vi "AR.Drone MAIN.vi"() -> ()   [LabVIEW 2014]
doc: "Very simple example showing how to use the base VIs to control the AR Drone and receive and display video data."
uses:
  Resources/Others/Control cluster.ctl
  <vilib>/LVH/AR Drone Toolkit/Decode NavData/Typedefs/NavData Demo.ctl
  Resources/Global.vi
  <vilib>/LVH/AR Drone Toolkit/AR Drone.lvlib
panel:
  in  "Tab Control 2":enum32{"Setup", "Debug&Test Info", "NavData"}(tab)
  in  "Secondary VI":u16(ring) items=["Auto Hovering with Position Prediction.vi", "Simple Video.vi", "Circle detection.vi", "OCR Control.vi", "", ""]
  in  "Setup Parameters":T1={"Drone IP address"="192.168.1.1", "Home IP address"="192.168.1.2", "Flight Mode"=enum."INDOOR MODE", "Mounted Hull"=enum."INDOOR HULL", "Video Camera"=1, "Max Altitude (m)"=3.0, "Max Pitch and Roll Angle (deg)"=8.0, "Max Vertical Speed (m/s)"=0.7, "Max Yaw Speed (deg/s)"=100.0} {"Video Camera" items=["Bottom Camera"=1, "Front Camera"=0, "Front in Bottom"=3, "Bottom in Front"=2]}
  in  "Controller ID":i32=2
  in  "Adjustments":cluster{"Sensitivity":dbl, "Null Zone":dbl}={"Sensitivity"=1.0, "Null Zone"=1.0} {"Null Zone" scale=0.0..2.0; "Sensitivity" scale=0.0..2.0}
  out "In. device":T2={"axes total"=0, "buttons total"=1280, "pov total"=0, "device name"="Micr"}
  out "Loop iteration":i32=255
  in  "milliseconds to wait":u32=10
  out "Refesh Rate (ms)":u32=10
  out "Refesh Rate Video Loop (ms) 2":u32=40
  in  "video refresh (ms)":u32=40
  out "Error":errorcluster
  out "NavData Out":T3={"control state"=enum."TRANS_LANDING", "battery percentage"=55, "pitch (deg)"=0.026, "roll (deg)"=-0.043, "yaw (deg)"=74.079, "altitude (cm)"=0, "vx (cm/s)?"=0.0, "vy (cm/s)?"=0.0, "vz (cm/s)?"=0.0, "detection cam type"=3}
  out "Battery Remaining":dbl(slide)=55.0 scale=0.0..100.0
  out "Hover":bool
  out "Control Cluster":T4 {"Yaw Speed" scale=-1.0..1.0; "Vertical Speed" scale=-1.0..1.0; "Pitch" scale=-1.0..1.0; "Roll" scale=-1.0..1.0}
  out "error":bool
  out "Take off/Land":bool
  in  "Tab Control":enum32{"Raw Image", "Grayscale", "Black&White"}(tab)=enum."Black&White"
  out "Raw":picture
  out "Grayscale":T5(plugin-control)
  out "B&W":T5(plugin-control)
  in  "Manual":bool=TRUE
  in  "stop":bool
  in  "Emergency Landing":bool
  # "(1 is default)"
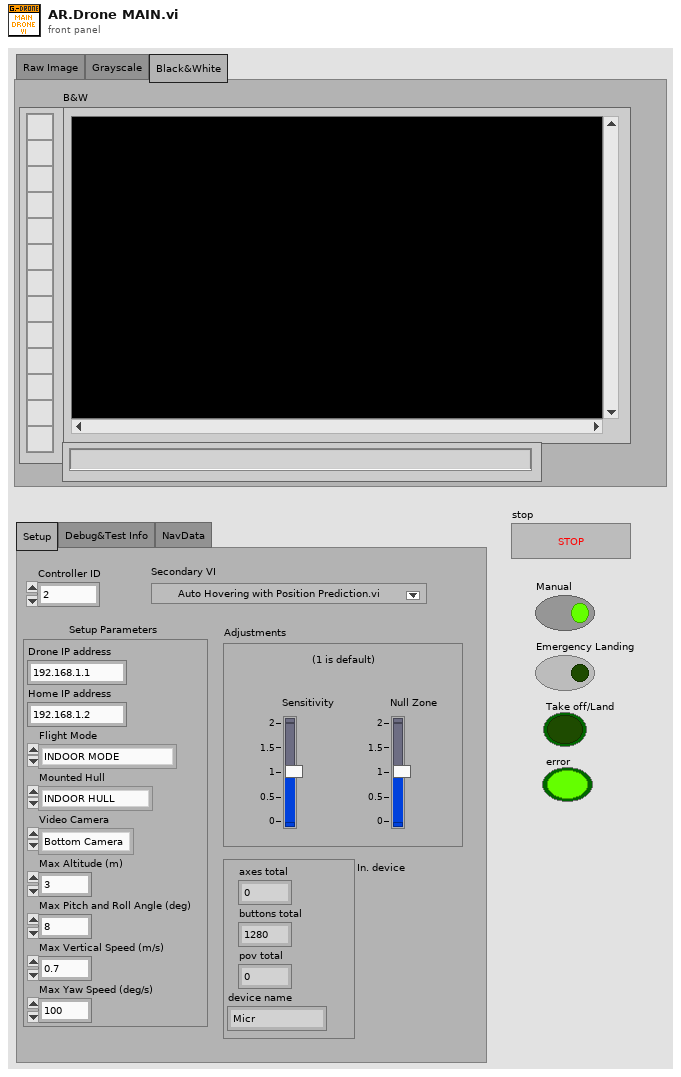
[diagram p1: front panel]
types:
  T1 = cluster{"Drone IP address":string, "Home IP address":string, "Flight Mode":enum8{"OUTDOOR MODE", "INDOOR MODE"}, "Mounted Hull":enum8{"OUTDOOR HULL", "INDOOR HULL"}, "Video Camera":u8, "Max Altitude (m)":sgl, "Max Pitch and Roll Angle (deg)":sgl, "Max Vertical Speed (m/s)":sgl, "Max Yaw Speed (deg/s)":sgl}
  T2 = cluster{"axes total":u32, "buttons total":u32, "pov total":u32, "device name":string}
  T3 = typedef "AR Drone.lvlib/NavData Demo.ctl" = cluster{"control state":enum32{"DEFAULT", "INIT", "LANDING", "FLYING", "HOVERING", "TEST", "TRANS_TAKEOFF", "TRANS_GOTOFIX", "TRANS_LANDING"}, "battery percentage":u32, "pitch (deg)":sgl, "roll (deg)":sgl, "yaw (deg)":sgl, "altitude (cm)":u32, "vx (cm/s)?":sgl, "vy (cm/s)?":sgl, "vz (cm/s)?":sgl, "detection cam type":u32}
  T4 = typedef "Control cluster.ctl" = cluster{"Roll":sgl, "Pitch":sgl, "Vertical Speed":sgl, "Yaw Speed":sgl}
  T5 = typedef "IMAQ Image.ctl" = refnum<image>
  T6 = typedef "AR Drone.lvlib/AR Drone Resource.ctl" = cluster{"UDP Control Connection":refnum<k16>, "UDP NavData Connection":refnum<k16>, "UDP Video Connection (Drone 1.0)":refnum<k16>, "TCP Video Connection (Drone 2.0)":refnum<k5>, "TCP Control Port Connection":refnum<k5>, "Drone IP address":string, "Drone Command Port":u16, "Drone NavData Port":u16, "Drone Vid Stream Port":u16, "Drone TCP Control Port":u16, "Home IP address":string, "Home Command Port":u16, "Home NavData Port":u16, "Home Vid Stream Port":u16, "Drone Version":i32, "Drone Index":i32, "Command Sequence":i32}
  T7 = cluster{"Roll":dbl, "Pitch":dbl, "Vertical Speed":dbl, "Yaw Speed":dbl}
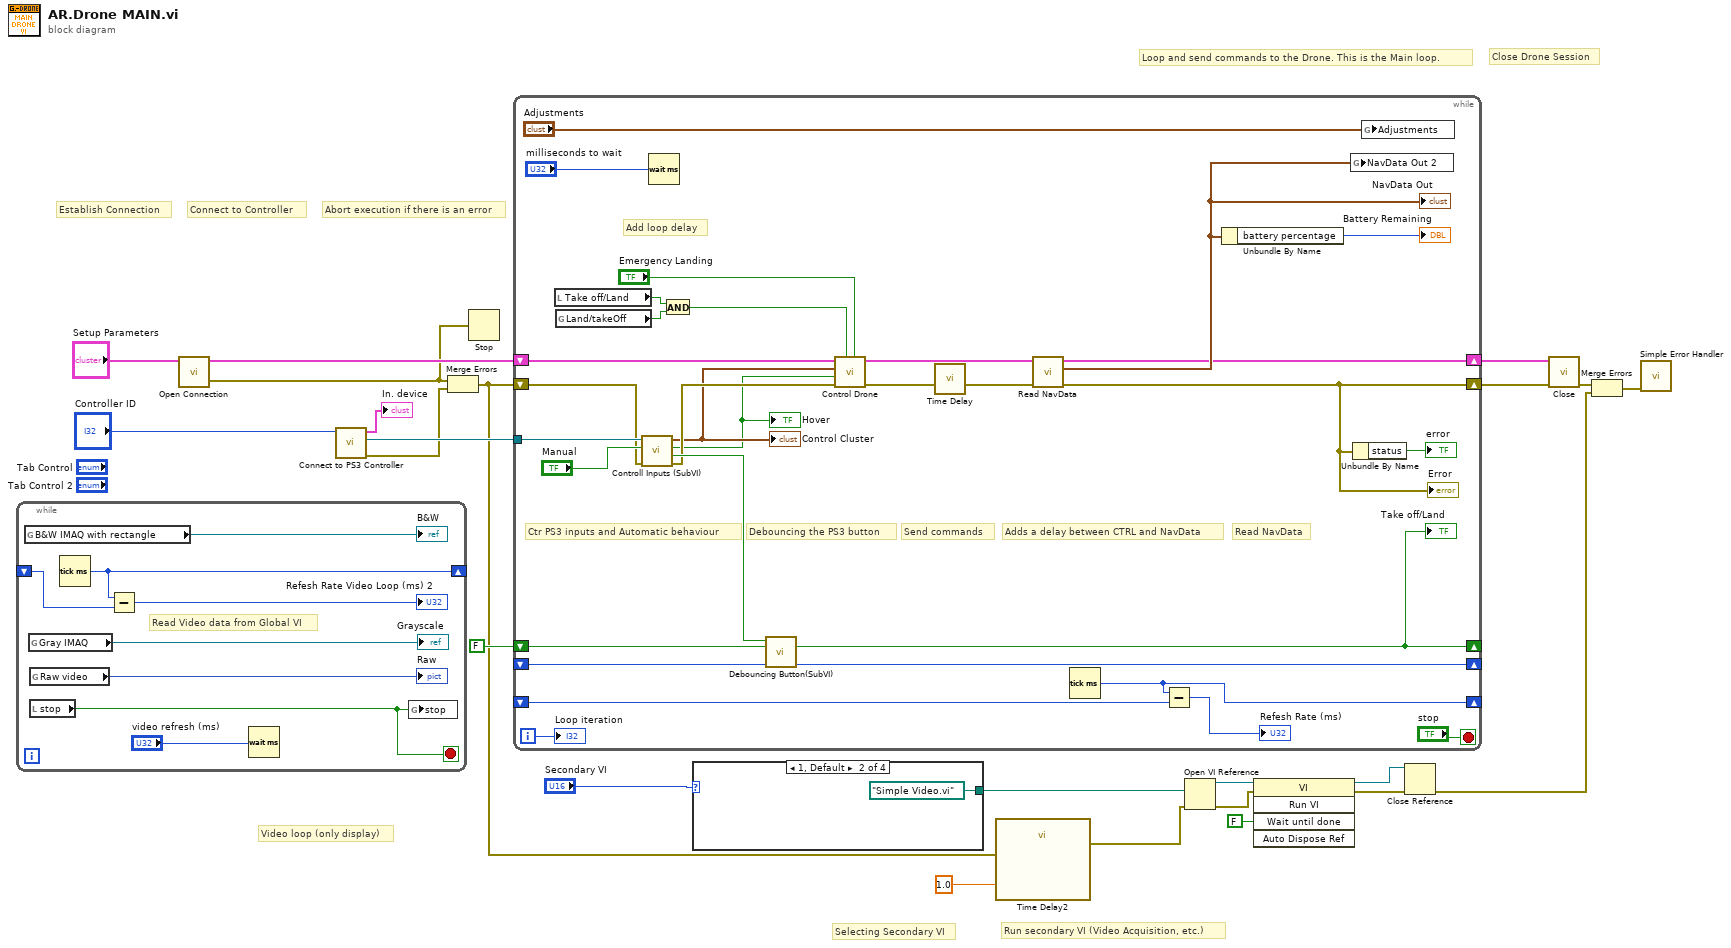
[diagram p0: block diagram]
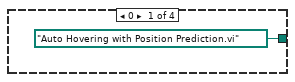
[diagram p2: hidden frame]
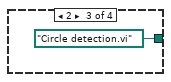
[diagram p3: hidden frame]
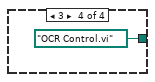
[diagram p4: hidden frame]
diagram:
  # "Selecting Secondary VI"
  # "Connect to Controller"
  # "Run secondary VI (Video Acquisition, etc.)"
  # "Abort execution if there is an error"
  # "Establish Connection"
  # "Video loop (only display)"
  # "Close Drone Session"
  # "Loop and send commands to the Drone. This is the Main loop."
  n1 = while {
    shift-right: [w25] -> _
    shift-left: _ -> [w30]
    stop <- w28 stop-if-true
    # "Read Video data from Global VI"
    n2 = global read "Global.vi" "B&W IMAQ with rectangle"() -> (→"B&W":T5)
    n3 = global read "Global.vi" "Gray IMAQ"() -> (→"Grayscale":T5)
    n4 = global read "Global.vi" "Raw video"() -> (→"Raw":picture)
    n5 = local read "stop"() -> (w28:bool)
    n6 = Tick Count (ms)() -> (millisecond timer value=w25:u32)
    n7 = Subtract(x=w25, y=w30) -> (x-y=→"Refesh Rate Video Loop (ms) 2":u32)
    n8 = Wait (ms)(milliseconds to wait="video refresh (ms)") -> ()  [unwired: 1 out]
    n9 = global write "Global.vi" "stop"(w28) -> ()
  }
  n10 = call "Open Connection.vi"("Setup Parameters"="Setup Parameters") -> ("error out"=w14:errorcluster, "AR Drone Resource"=w20:T6)  [unwired: 9 in]
  n11 = call "Connect to PS3 Controller.vi"("device ID"="Controller ID") -> ("error out"=w13:errorcluster, "device ID 2"=w17:refnum<k1>, "element"=→"In. device":T2)  [unwired: 7 in]
  n12 = Merge Errors(w14, w13) -> (w5:errorcluster)
  n13 = Stop(stop? (T)=w14) -> ()
  n14 = while {
    shift-right: [w43] -> w23
    shift-left: w20 -> [w61]
    shift-right: [w39] -> w21
    shift-left: w5 -> [w38]
    shift-right: [w35] -> _
    shift-left: _ -> [w56]
    shift-right: [w53] -> _
    shift-left: FALSE -> [w54]
    shift-right: [w52] -> _
    shift-left: _ -> [w51]
    tunnel: w17 -> [w45]
    i -> [w60]
    stop <- "stop" stop-if-true
    # "Add loop delay"
    # "Ctr PS3 inputs and Automatic behaviour"
    # "Read NavData"
    # "Send commands"
    # "Debouncing the PS3 button"
    # "Adds a delay between CTRL and NavData"
    n15 = local read "Take off/Land"() -> (w33:bool)
    n16 = global read "Global.vi" "Land/takeOff"() -> (w34:bool)
    n17 = call "Controll Inputs (SubVI).vi"("error in (no error)"=w38, "Manual"="Manual", "Refnum in"=w45) -> ("error out"=w37:errorcluster, "Land/Take off"=w55:bool, "Boolean"=w32:bool, "Control cluster"=w36:T7)  [unwired: 5 in]
    "Control Cluster" <- w36
    "Hover" <- w32
    n18 = Wait (ms)(milliseconds to wait="milliseconds to wait") -> ()  [unwired: 1 out]
    n19 = And(x=w33, y=w34) -> (x .and. y?=w46:bool)
    n20 = call "Debouncing Button(SubVI).vi"("millisecond timer value in"=w51, "Boolean in"=w54, "Land/Take off"=w55) -> ("millisecond timer value out"=w52:u32, "Boolean out"=w53:bool)  [unwired: 7 in]
    "Take off/Land" <- w53
    n21 = call <vilib>:"Control Drone.vi"("Emergency Landing"="Emergency Landing", "Takeoff/Land"=w46, "error in (no error)"=w37, "Hover"=w32, "Control Cluster"=w36, "AR Drone Resource"=w61) -> ("error out"=w41:errorcluster, "AR Drone Resource Out"=w59:T6)  [unwired: 4 in]
    n22 = call "Time Delay"("error in (no error)"=w41) -> ("error out"=w42:errorcluster)  [unwired: 10 in]
    n23 = call <vilib>:"Read NavData.vi"("error in (no error)"=w42, "AR Drone Resource"=w59) -> ("error out"=w39:errorcluster, "NavData Out"=w48:T3, "AR Drone Resource Out"=w43:T6)  [unwired: 7 in]
    "Error" <- w39
    "NavData Out" <- w48
    n24 = Tick Count (ms)() -> (millisecond timer value=w35:u32)
    n25 = Subtract(x=w35, y=w56) -> (x-y=→"Refesh Rate (ms)":u32)
    n26 = Unbundle By Name(w48) -> ("battery percentage"=→"Battery Remaining":u32)
    n27 = global write "Global.vi" "NavData Out 2"(w48) -> ()
    n28 = Unbundle By Name(w39) -> ("status"=→"error":bool)
    n29 = global write "Global.vi" "Adjustments"("Adjustments") -> ()
    "Loop iteration" <- w60
  }
  n30 = case shown="1, Default" "Secondary VI" {
    tunnel: [path "Auto Hovering with Position Prediction.vi" ("Video Acquisition VI path") path "Simple Video.vi" ("Video Acquisition VI path") path "Circle detection.vi" ("Video Acquisition VI path") path "OCR Control.vi" ("Video Acquisition VI path")] -> w10
    frame 0 {
    }
    frame 1, Default {
    }
    frame 2 {
    }
    frame 3 {
    }
  }
  n31 = call "Time Delay2"("error in (no error)"=w5, "Delay Time (s)"=1.0) -> ("error out"=w11:errorcluster)  [unwired: 9 in]
  n32 = Open VI Reference(vi path=w10, error in (no error)=w11) -> (vi reference=w8:refnum<vi>, error out=w6:errorcluster)  [unwired: 4 in]
  n33 = invoke class="VI" method="Run VI"(reference=w8, error in=w6, "Wait until done"=FALSE) -> (reference out=w7:refnum<vi>, error out=w12:errorcluster)  [unwired: 2 in, 3 out]
  n34 = Close Reference(reference=w7, error in (no error)=w12) -> (error out=w1:errorcluster)
  n35 = call <vilib>:"Close.vi"("error in (no error)"=w21, "AR Drone Resource"=w23) -> ("error out"=w2:errorcluster)  [unwired: 9 in]
  n36 = Merge Errors(w2, w1) -> (w19:errorcluster)
  n37 = call <vilib>:"Simple Error Handler.vi"("error in (no error)"=w19) -> ()  [unwired: 4 in, 5 out]
